vi "ziGetCurrentCalcVec.vi"(4 "Gain (), Shunt (ohm)":dbl, 5 "VGain":dbl, 6 "Imp50 (F)":bool, 7 "R":dbl, 10 "DemodVoltage (Vrms)":cdb[](array[numeric]) format="%#_6p", 11 "Mode":T1(ring)) -> (2 "I (Arms)":cdb[](array[numeric]) format="%#_6p")   [LabVIEW 2018, in "Zurich Instruments LabOne.lvlib"]
uses:
  Zurich Instruments LabOne.lvlib
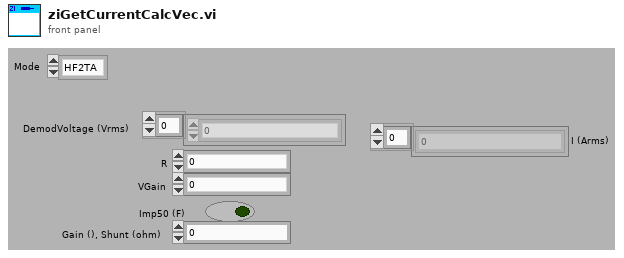
[diagram p1: front panel]
types:
  T1 = enum16{"HF2TA", "HF2CA", "Int. Shunt", "Ext. Shunt"}
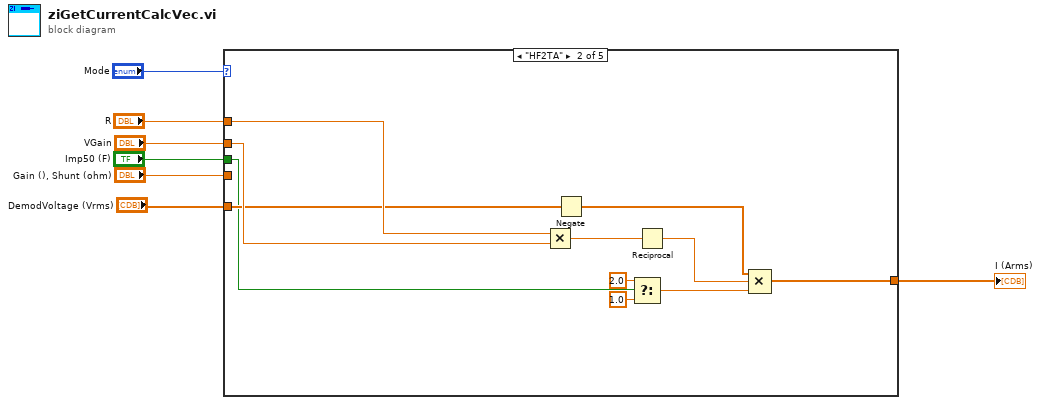
[diagram p0: block diagram]
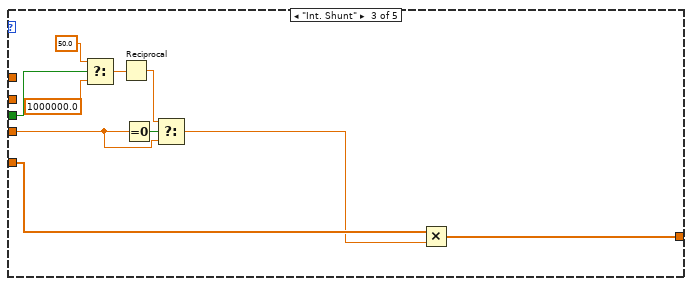
[diagram p3: hidden frame]
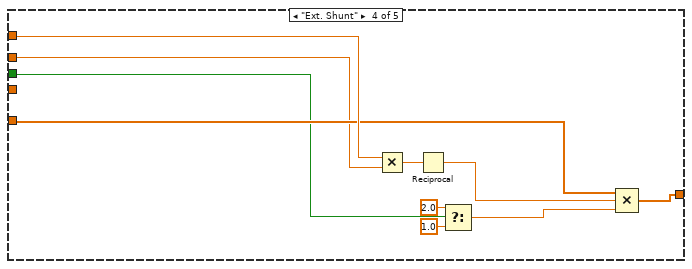
[diagram p4: hidden frame]
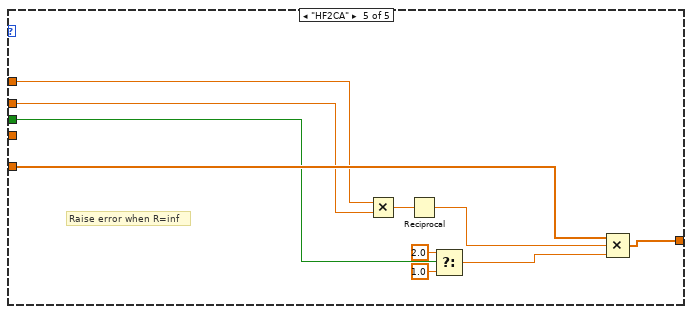
[diagram p5: hidden frame]
diagram:
  n1 = case shown="\"HF2TA\"" "Mode" {
    tunnel: "VGain" -> [_ w14 _ w31 w43]
    tunnel: "Imp50 (F)" -> [_ w8 w19 w29 w39]
    tunnel: [_ w11 w28 w30 w44] -> w3
    tunnel: "R" -> [_ w15 _ w33 w42]
    tunnel: "DemodVoltage (Vrms)" -> [_ w10 w27 w32 w45]
    tunnel: "Gain (), Shunt (ohm)" -> [_ _ w25 _ _]
    frame Default {
    }
    frame "HF2TA" {
      n2 = Multiply(x=w15, y=w14) -> (x*y=w13:dbl)
      n3 = Negate(x=w10) -> (-x=w9:cdb[])
      n4 = Select(t=2.0, s=w8, f=1.0) -> (s? t:f=w16:dbl)
      n5 = Reciprocal(x=w13) -> (1/x=w12:dbl)
      n6 = Compound Arithmetic op=MULTIPLY(w9, w12, w16) -> (w11:cdb[])
    }
    frame "Int. Shunt" {
      n7 = Select(t=50.0 ("f"), s=w19, f=1000000.0 ("t")) -> (s? t:f=w24:dbl)
      n8 = Reciprocal(x=w24) -> (1/x=w23:dbl)
      n9 = Equal To 0?(x=w25) -> (x = 0?=w26:bool)
      n10 = Select(t=w23, s=w26, f=w25) -> (s? t:f=w22:dbl)
      n11 = Multiply(x=w27, y=w22) -> (x*y=w28:cdb[])
    }
    frame "Ext. Shunt" {
      n12 = Multiply(x=w33, y=w31) -> (x*y=w37:dbl)
      n13 = Reciprocal(x=w37) -> (1/x=w38:dbl)
      n14 = Select(t=2.0, s=w29, f=1.0) -> (s? t:f=w36:dbl)
      n15 = Compound Arithmetic op=MULTIPLY(w32, w38, w36) -> (w30:cdb[])
    }
    frame "HF2CA" {
      # "Raise error when R=inf"
      n16 = Multiply(x=w42, y=w43) -> (x*y=w41:dbl)
      n17 = Reciprocal(x=w41) -> (1/x=w40:dbl)
      n18 = Select(t=2.0, s=w39, f=1.0) -> (s? t:f=w46:dbl)
      n19 = Compound Arithmetic op=MULTIPLY(w45, w40, w46) -> (w44:cdb[])
    }
  }
  "I (Arms)" <- w3
